vi "Async.vi"(11 "Async Data":T1={"Hardware"={"Switch Device"="", "DMM Device"="PXI1Slot6", "DMM -> Switch Trigger"=0, "Switch -> DMM Trigger"=0, "Sample Interval (sec)"=0.1, "Current Samples"=1, "Current Limit"=1.2, "Current Resolution"=5.5, "Auto-Read"=FALSE, "Keep Values"=FALSE}, "Communication"={"Status Q"=refnum, "Command Q"=refnum, "Voltage FIFO"=refnum, "Voltage Buffer"=[], "Current FIFO"=refnum, "Current Buffer"=[], "Async Events"=refnum}} {"Hardware"."Current Resolution" items=["3 1/2"=3.5, "4 1/2"=4.5, "5 1/2"=5.5, "6 1/2"=6.5, "7 1/2"=7.5]; "Hardware"."Sample Interval (sec)" format="%.2f"}) -> ()   [LabVIEW 2011, in "Switch-DMM Custom Device.lvlib"]
uses:
  Switch-DMM Custom Device.lvlib
  Controls/Async Data.ctl
  Controls/Hardware.ctl
  <instrlib>/niDMM/nidmm.llb/niDMM Resolution in Digits.ctl
  Controls/Communication.ctl
  Controls/Async Status.ctl
  Controls/Async State.ctl
  Controls/Async Command.ctl
  Controls/Async Events.ctl
  Controls/Cur Loop Cmd.ctl
panel:
  out "error out":errorcluster
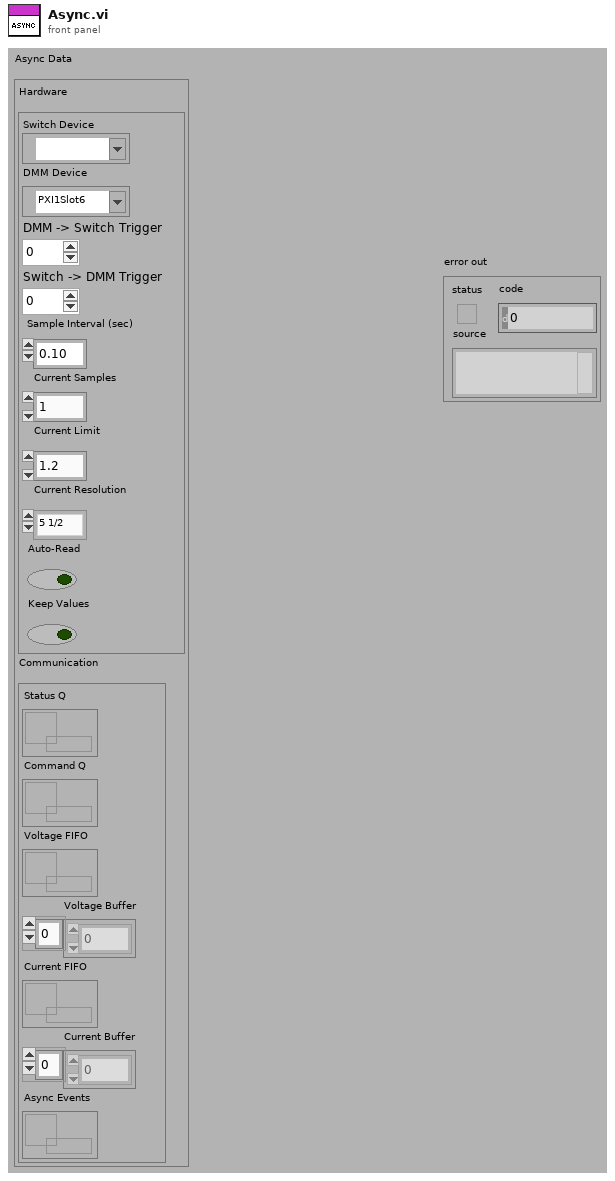
[diagram p1: front panel]
types:
  T1 = typedef "Switch-DMM Custom Device.lvlib/Async Data.ctl" = cluster{"Hardware":T2, "Communication":T4}
  T2 = typedef "Switch-DMM Custom Device.lvlib/Hardware.ctl" = cluster{"Switch Device":refnum<k15>, "DMM Device":refnum<k15>, "DMM -> Switch Trigger":u16, "Switch -> DMM Trigger":u16, "Sample Interval (sec)":dbl, "Current Samples":i32, "Current Limit":dbl, "Current Resolution":T3, "Auto-Read":bool, "Keep Values":bool}
  T3 = typedef "niDMM Resolution in Digits.ctl" = dbl
  T4 = typedef "Switch-DMM Custom Device.lvlib/Communication.ctl" = cluster{"Status Q":refnum<queue>, "Command Q":refnum<queue>, "Voltage FIFO":refnum<k33>, "Voltage Buffer":dbl[], "Current FIFO":refnum<k33>, "Current Buffer":dbl[], "Async Events":refnum<queue>}
  T5 = typedef "Switch-DMM Custom Device.lvlib/Async State.ctl" = enum16{"Not running", "Initializing", "Waiting on start cmd", "Running", "Stopped"}
  T6 = typedef "Switch-DMM Custom Device.lvlib/Async Command.ctl" = enum16{"None", "Start", "Set Cur Mode", "Req Volt Mode", "Set Volt Mode", "Read Volt", "Exit"}
  T7 = typedef "Switch-DMM Custom Device.lvlib/Cur Loop Cmd.ctl" = enum16{"None", "Start", "Stop", "Exit"}
  T8 = typedef "Bosch Switch-DMM Custom Device.lvlib/Cur Loop Cmd.ctl" = enum16{"None", "Start", "Stop", "Exit"}
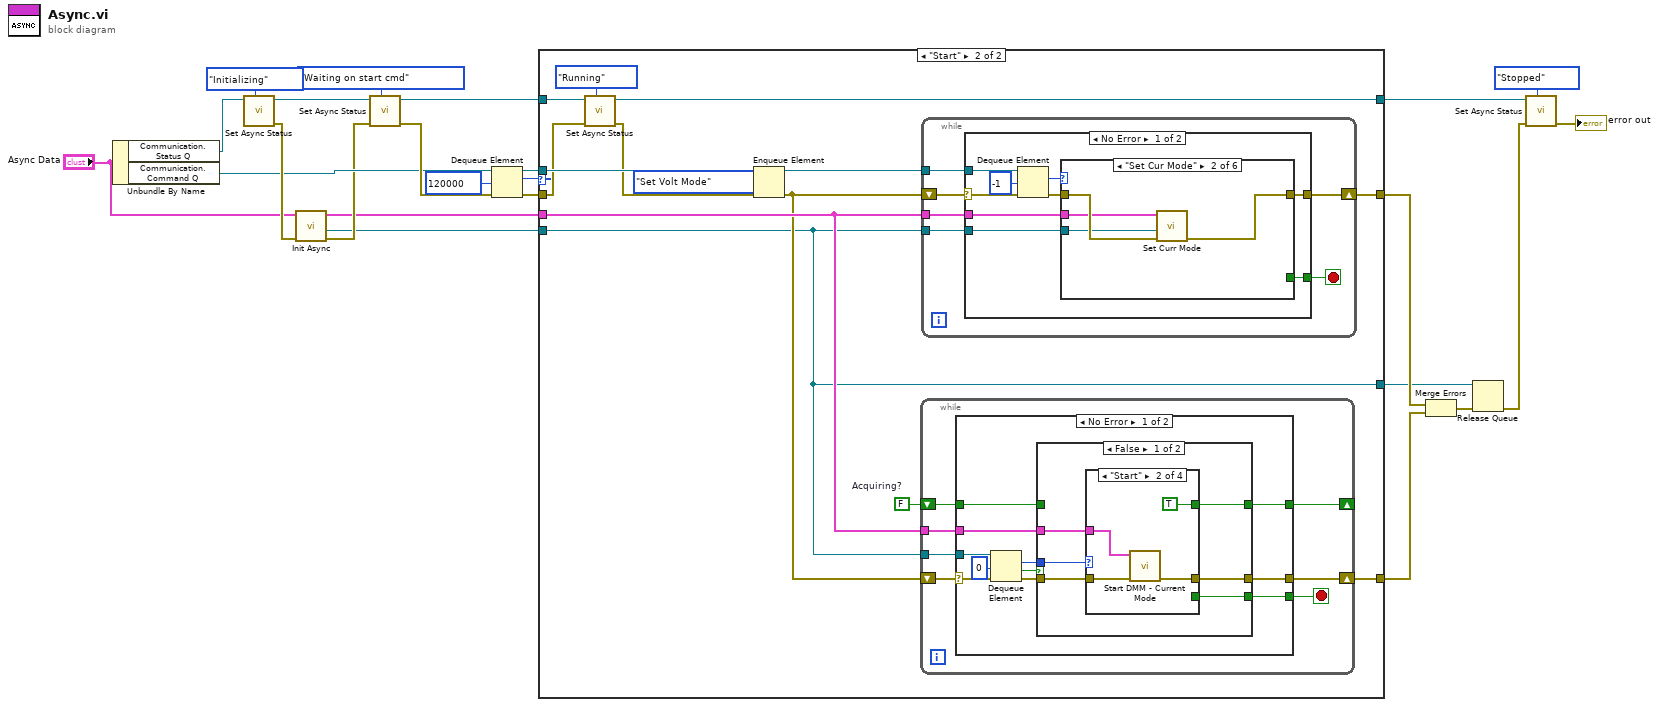
[diagram p0: block diagram]
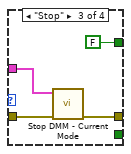
[diagram p4: hidden frame]
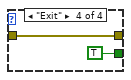
[diagram p5: hidden frame]
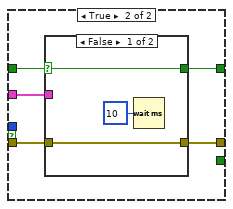
[diagram p6: hidden frame]
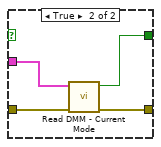
[diagram p7: hidden frame]
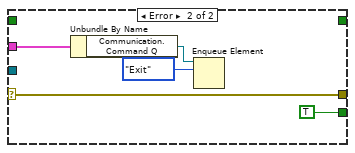
[diagram p8: hidden frame]
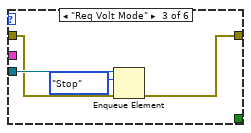
[diagram p10: hidden frame]
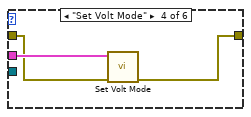
[diagram p11: hidden frame]
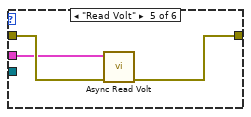
[diagram p12: hidden frame]
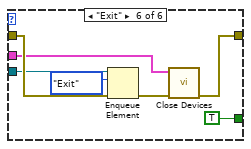
[diagram p13: hidden frame]
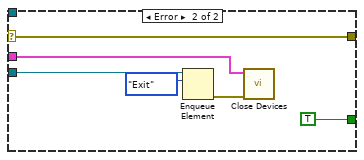
[diagram p14: hidden frame]
diagram:
  n1 = Unbundle By Name("Async Data") -> ("Communication.Status Q"=w24:refnum<queue>, "Communication.Command Q"=w7:refnum<queue>)
  n2 = call "Set Async Status.vi"("State"=Async_State."Initializing", "queue in"=w24) -> ("error out"=w14:errorcluster, "queue out"=w22:refnum<queue>)  [unwired: 8 in]
  n3 = call "Init Async.vi"("error in (no error)"=w14, "Async Data in"="Async Data") -> ("error out"=w6:errorcluster, "Cur Loop Cmd Q"=w4:refnum<queue>, "Async Data out"=w5:T1)  [unwired: 7 in]
  n4 = call "Set Async Status.vi"("State"=Async_State."Waiting on start cmd", "error in (no error)"=w6, "queue in"=w22) -> ("error out"=w19:errorcluster, "queue out"=w16:refnum<queue>)  [unwired: 7 in]
  n5 = Dequeue Element(queue=w7, timeout in ms (-1)=120000, error in (no error)=w19) -> (queue out=w15:refnum<queue>, element=w18:T6, error out=w17:errorcluster)  [unwired: 1 out]
  n6 = case shown="\"Start\"" w18 {
    tunnel: w17 -> [w26 w37]
    tunnel: w16 -> [w27 w38]
    tunnel: w15 -> [_ w41]
    tunnel: [w27 w35] -> w11
    tunnel: [w26 w40] -> w10
    tunnel: [_ w39] -> w9
    tunnel: w5 -> [_ w33]
    tunnel: w4 -> [w25 w28]
    tunnel: [w25 w28] -> w1
    frame "None", Default {
    }
    frame "Start" {
      w29 = FALSE  # Acquiring?
      n7 = call "Set Async Status.vi"("State"=Async_State."Running", "error in (no error)"=w37, "queue in"=w38) -> ("error out"=w36:errorcluster, "queue out"=w35:refnum<queue>)  [unwired: 7 in]
      n8 = Enqueue Element(queue=w41, element=Async_Command."Set Volt Mode" ("Async Command"), error in (no error)=w36) -> (queue out=w31:refnum<queue>, error out=w30:errorcluster)  [unwired: 1 in, 1 out]
      n9 = while {
        shift-right: [w44] -> w39
        shift-left: w30 -> [w42]
        tunnel: w28 -> [w48]
        tunnel: w33 -> [w47]
        shift-right: [w45] -> _
        shift-left: w29 -> [w46]
        stop <- w43 stop-if-true
        n10 = case shown="No Error" w42 {
          selector: w42 -> [w49 w92]
          tunnel: w48 -> [w58 _]
          tunnel: w47 -> [w54 w90]
          tunnel: w46 -> [w53 _]
          tunnel: [w52 _] -> w45
          tunnel: [w51 w92] -> w44
          tunnel: [w50 TRUE] -> w43
          frame No Error {
            n11 = Dequeue Element(queue=w58, timeout in ms (-1)=0, error in (no error)=w49) -> (element=w56:T8, timed out?=w57:bool, error out=w55:errorcluster)  [unwired: 1 out]
            n12 = case shown="False" w57 {
              tunnel: w56 -> [w65 _]
              tunnel: w55 -> [w64 w80]
              tunnel: w54 -> [w63 w79]
              tunnel: w53 -> [_ w81]
              tunnel: [w62 w78] -> w52
              tunnel: [w61 w77] -> w51
              tunnel: [w60 _] -> w50
              frame False {
                n13 = case shown="\"Start\"" w65 {
                  tunnel: w64 -> [w66 w69 w72 w76]
                  tunnel: w63 -> [_ w70 w73 _]
                  tunnel: [_ TRUE ("Acquiring?") FALSE ("Acquiring?") _] -> w62
                  tunnel: [w66 w67 w71 w76] -> w61
                  tunnel: [_ _ _ TRUE] -> w60
                  frame "None", Default {
                  }
                  frame "Start" {
                    n14 = call "Start DMM - Current Mode.vi"("error in (no error)"=w69, "Async Data out"=w70) -> ("error out"=w67:errorcluster)  [unwired: 9 in]
                  }
                  frame "Stop" {
                    n15 = call "Stop DMM - Current Mode.vi"("error in (no error)"=w72, "Async Data out"=w73) -> ("error out"=w71:errorcluster)  [unwired: 9 in]
                  }
                  frame "Exit" {
                  }
                }
              }
              frame True {
                n16 = case shown="False" w81 {
                  selector: w81 -> [w83 _]
                  tunnel: w80 -> [w82 w87]
                  tunnel: w79 -> [_ w88]
                  tunnel: [w83 w86] -> w78
                  tunnel: [w82 w85] -> w77
                  frame False {
                    n17 = Wait (ms)(milliseconds to wait=u32 10) -> ()  [unwired: 1 out]
                  }
                  frame True {
                    n18 = call "Read DMM - Current Mode.vi"("error in (no error)"=w87, "Async Data in"=w88) -> ("error out"=w85:errorcluster, "Acquiring"=w86:bool)  [unwired: 8 in]
                  }
                }
              }
            }
          }
          frame Error {
            n19 = Unbundle By Name(w90) -> ("Communication.Command Q"=w89:refnum<queue>)
            n20 = Enqueue Element(queue=w89, element=Async_Command."Exit") -> ()  [unwired: 2 in, 3 out]
          }
        }
      }
      n21 = while {
        tunnel: w31 -> [w99]
        shift-right: [w95] -> w40
        shift-left: w30 -> [w94]
        tunnel: w33 -> [w97]
        tunnel: w28 -> [w96]
        stop <- w98 stop-if-true
        n22 = case shown="No Error" w94 {
          selector: w94 -> [w100 w132]
          tunnel: w99 -> [w108 _]
          tunnel: [w104 TRUE] -> w98
          tunnel: w97 -> [w103 w134]
          tunnel: w96 -> [w102 w135]
          tunnel: [w101 w132] -> w95
          frame No Error {
            n23 = Dequeue Element(queue=w108, timeout in ms (-1)=-1, error in (no error)=w100) -> (element=w107:T6, error out=w105:errorcluster)  [unwired: 2 out]
            n24 = case shown="\"Set Cur Mode\"" w107 {
              tunnel: w105 -> [w109 w113 w115 w119 w123 w129]
              tunnel: [_ _ _ _ _ TRUE] -> w104
              tunnel: w103 -> [_ w111 _ w120 w122 w126]
              tunnel: w102 -> [_ w110 w117 _ _ w128]
              tunnel: [w109 w112 w114 w118 w121 w124] -> w101
              frame "None", Default {
              }
              frame "Set Cur Mode" {
                n25 = call "Set Curr Mode.vi"("error in (no error)"=w113, "Curr Loop Cmd Q"=w110, "Async Data in"=w111) -> ("error out"=w112:errorcluster)  [unwired: 8 in]
              }
              frame "Req Volt Mode" {
                n26 = Enqueue Element(queue=w117, element=Cur_Loop_Cmd."Stop", error in (no error)=w115) -> (error out=w114:errorcluster)  [unwired: 1 in, 2 out]
              }
              frame "Set Volt Mode" {
                n27 = call "Set Volt Mode.vi"("error in (no error)"=w119, "Async Data in"=w120) -> ("error out"=w118:errorcluster)  [unwired: 9 in]
              }
              frame "Read Volt" {
                n28 = call "Async Read Volt.vi"("error in (no error)"=w123, "Async Data out"=w122) -> ("error out"=w121:errorcluster)  [unwired: 9 in]
              }
              frame "Exit" {
                n29 = Enqueue Element(queue=w128, element=Cur_Loop_Cmd."Exit", error in (no error)=w129) -> (error out=w125:errorcluster)  [unwired: 1 in, 2 out]
                n30 = call "Close Devices.vi"("error in (no error)"=w125, "Async Data out"=w126) -> ("error out"=w124:errorcluster)  [unwired: 9 in]
              }
            }
          }
          frame Error {
            n31 = Enqueue Element(queue=w135, element=Cur_Loop_Cmd."Exit") -> (error out=w133:errorcluster)  [unwired: 2 in, 2 out]
            n32 = call "Close Devices.vi"("error in (no error)"=w133, "Async Data out"=w134) -> ()  [unwired: 9 in, 1 out]
          }
        }
      }
    }
  }
  n33 = Merge Errors(w10, w9) -> (w3:errorcluster)
  n34 = Release Queue(queue=w1, error in (no error)=w3) -> (error out=w2:errorcluster)  [unwired: 1 in, 2 out]
  n35 = call "Set Async Status.vi"("State"=Async_State."Stopped", "error in (no error)"=w2, "queue in"=w11) -> ("error out"=→"error out":errorcluster)  [unwired: 7 in, 1 out]
